vi "Game_PackStateForUI.vi"(7 "Puzzle State":string, 8 "error in (no error)":errorcluster, 9 "Can Buy Vowel?":bool, 10 "player":T2, 11 "Players array":T3[](array[typedef])) -> (0 "error out":errorcluster, 3 "gameState":T1)   [LabVIEW 2020]
uses:
  Typedefs/game_player.ctl
  Typedefs/enumeratedPlayers.ctl
  Typedefs/gameState.ctl
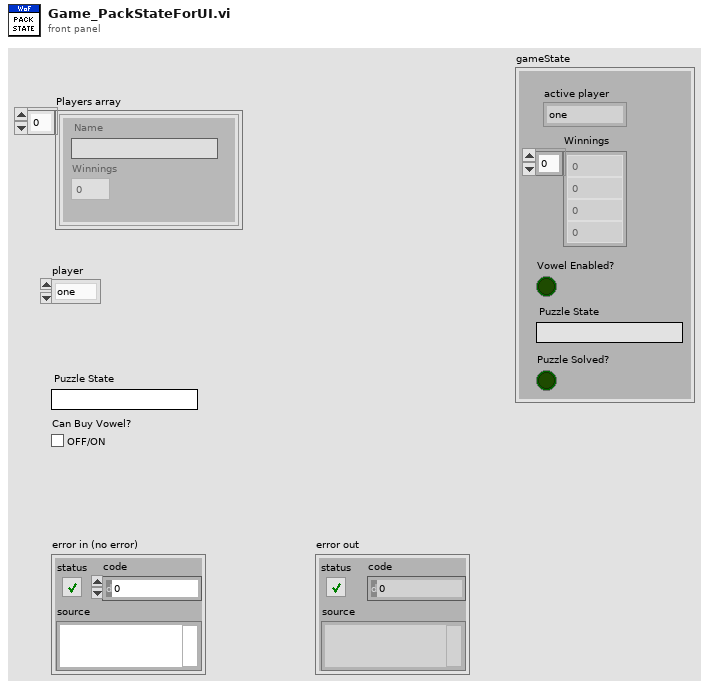
[diagram p1: front panel]
types:
  T1 = typedef "gameState.ctl" = cluster{"active player":T2, "Winnings":dbl[], "Vowel Enabled?":bool, "Puzzle State":string, "Puzzle Solved?":bool}
  T2 = typedef "enumeratedPlayers.ctl" = enum16{"one", "two", "three"}
  T3 = typedef "game_player.ctl" = cluster{"Name":string, "Winnings":dbl}
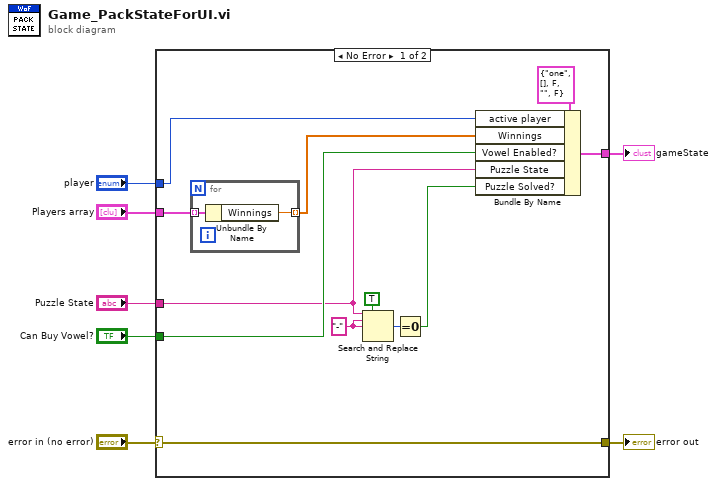
[diagram p0: block diagram]
diagram:
  n1 = case shown="No Error" "error in (no error)" {
    selector: "error in (no error)" -> [w9 w22]
    tunnel: "Can Buy Vowel?" -> [w15 _]
    tunnel: "Players array" -> [w17 _]
    tunnel: "Puzzle State" -> [w11 _]
    tunnel: "player" -> [w18 _]
    tunnel: [w9 w22] -> w2
    tunnel: [w8 _] -> w1
    frame No Error {
      w12 = "-" ("search string")
      n2 = for {
        tunnel: w17 -> [w21] mode=indexing
        tunnel: [w20] -> w16 mode=indexing
        n3 = Unbundle By Name(w21) -> ("Winnings"=w20:dbl)
      }
      n4 = Search and Replace String(replace all?=TRUE ("replace all? (F)"), input string=w11, search string=w12, replace string=w12) -> (number of replacements=w14:i32)  [unwired: 4 in, 3 out]
      n5 = Equal To 0?(x=w14) -> (x = 0?=w10:bool)
      n6 = Bundle By Name(cluster=T1 {"active player"=enum."one", "Winnings"=[], "Vowel Enabled?"=FALSE, "Puzzle State"="", "Puzzle Solved?"=FALSE} ("gameState"), "active player"=w18, "Winnings"=w16, "Vowel Enabled?"=w15, "Puzzle State"=w11, "Puzzle Solved?"=w10) -> (w8:T1)
    }
    frame Error {
    }
  }
  "error out" <- w2
  "gameState" <- w1
